vi "Write Source.vi"(8 "error in (no error)":errorcluster, 10 "Source":T3, 11 "Target in":refnum<class "Target.lvclass">) -> (0 "error out":errorcluster, 3 "Target out":refnum<class "Target.lvclass">)   [LabVIEW 2015, in "Target.lvclass"]
uses:
  Target.lvclass
  XML Controls/Path Cluster.ctl
  XML Controls/Supported Targets.ctl
  Target.lvclass/Target.ctl
  VeriStand Custom Device XML Parser.lvlib
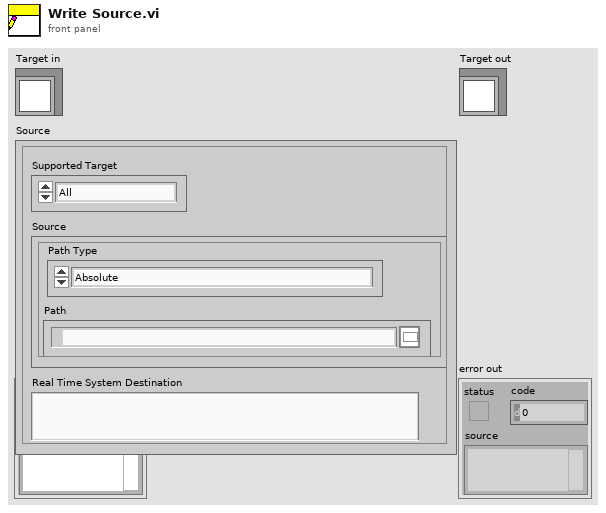
[diagram p1: front panel]
types:
  T1 = typedef "VeriStand Custom Device XML Parser.lvlib/Path Cluster.ctl" = cluster{"Path":path, "Path Type":enum16{"Absolute", "To Base", "To Common Doc Dir", "To Application Data Dir"}}
  T2 = typedef "VeriStand Custom Device XML Parser.lvlib/Supported Targets.ctl" = enum16{"All", "Pharlap", "VxWorks", "Windows", "Linux_32_ARM", "Linux_x64", "PharlapWindows", "PharlapVxWorks", "VxWorksWindows"}
  T3 = cluster{"Source":T1, "Real Time System Destination":string, "Supported Target":T2}
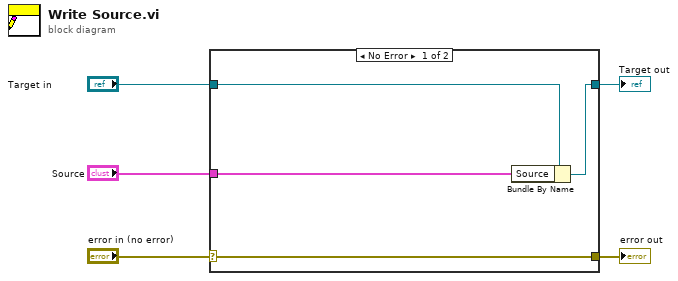
[diagram p0: block diagram]
diagram:
  n1 = case shown="No Error" "error in (no error)" {
    selector: "error in (no error)" -> [w9 w10]
    tunnel: [w9 w10] -> w4
    tunnel: [w7 w11] -> w2
    tunnel: "Target in" -> [w8 w11]
    tunnel: "Source" -> [w6 _]
    frame No Error {
      n2 = Bundle By Name(cluster=w8, "Source"=w6) -> (w7:refnum<class "Target.lvclass">)
    }
    frame Error {
    }
  }
  "error out" <- w4
  "Target out" <- w2
